vi "Execute.vi"(8 "error in":errorcluster, 11 "Change Flow in":refnum<class "Change Flow.lvclass">) -> (0 "error out":errorcluster, 1 "Next Step?":bool, 2 "MSG":string, 3 "Change Flow out":refnum<class "Change Flow.lvclass">)   [LabVIEW 2015, in "Change Flow.lvclass"]
uses:
  Change Flow.lvclass
  Reusable/Sequence/STEPS/LEAVES/Double/Switch DBL.lvclass/Switch DBL.ctl
  Reusable/Sequence/STEPS/LEAVES/Double/Read val.vi
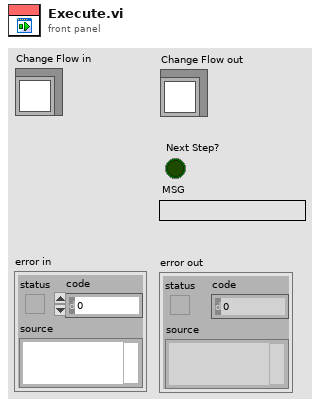
[diagram p1: front panel]
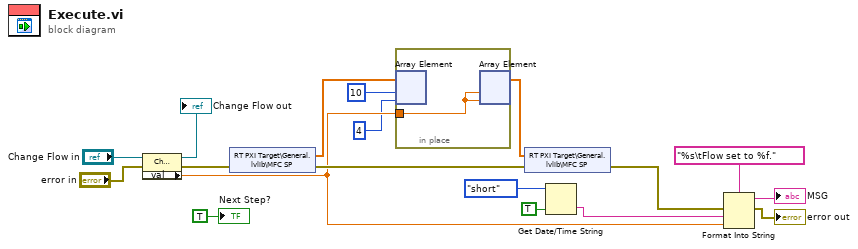
[diagram p0: block diagram]
diagram:
  n1 = property class="Change Flow"(reference="Change Flow in", error in="error in") -> (reference out=→"Change Flow out":refnum<class "Change Flow.lvclass">, error out=w11:errorcluster, "val"=w4:dbl)
  n2 = shared-variable "RT PXI Target\\General.lvlib\\MFC SP"(error in=w11) -> (w12:sgl[], error out=w14:errorcluster)
  n3 = in-place {
    in-place-border: w4 -> [w19]
    n4 = in-place-array #1(w12, 10 ("index"), 4) -> ()  [unwired: 2 out]
    n5 = in-place-array #1(w19, w19) -> (w10:sgl[])  [unwired: 2 out]
  }
  n6 = shared-variable "RT PXI Target\\General.lvlib\\MFC SP"(w10, error in=w14) -> (error out=w2:errorcluster)
  n7 = Get Date/Time String(date format (0)=enum16{"short", "long", "abbreviated"}."short", want seconds? (F)=TRUE) -> (time string=w7:string)  [unwired: 1 in, 1 out]
  n8 = Format Into String(format string="%s\tFlow set to %f.", error in=w2, w7, w4) -> (resulting string=→"MSG":string, error out=→"error out":errorcluster)  [unwired: 1 in]
  "Next Step?" <- TRUE ("Next Step?")
